vi "15-LeastRiskyPath.vi"(9 "position":cluster{"Row":i32, "Col":i32}, 10 "map in":T1(c390)) -> (2 "Min Risk":i32)   [LabVIEW 2019, in "15.lvlib"]
uses:
  15.lvlib
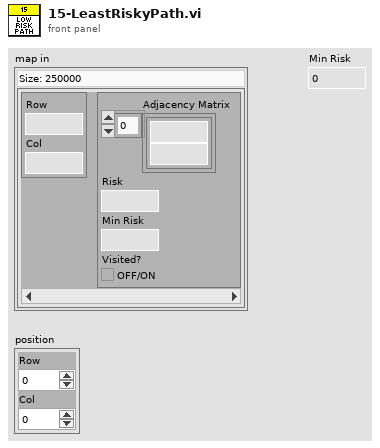
[diagram p1: front panel]
types:
  T1 = map{cluster{"Row":i32, "Col":i32}, cluster{"Adjacency Matrix":cluster{i32, i32}[], "Risk":u8, "Min Risk":i32, "Visited?":bool}}
  T2 = cluster{"Adjacency Matrix":cluster{i32, i32}[], "Risk":u8, "Min Risk":i32, "Visited?":bool}
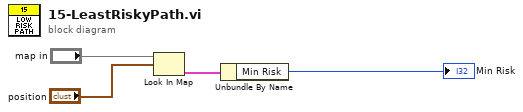
[diagram p0: block diagram]
diagram:
  n1 = Look In Map(map="map in", key="position") -> (value=w2:T2)  [unwired: 1 in, 1 out]
  n2 = Unbundle By Name(w2) -> ("Min Risk"=→"Min Risk":i32)
